vi "aal_moving average with decimation by order (real input).vi"(1 "Reset":bool, 2 "N":i32=2, 3 "x":dbl[](array[numeric])) -> (0 "y":dbl[](array[numeric]))   [LabVIEW 2014, in "NI_AALPro.lvlib"]
uses:
  NI_AALPro.lvlib
  lvanlys.dll
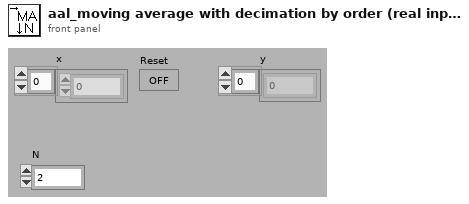
[diagram p1: front panel]
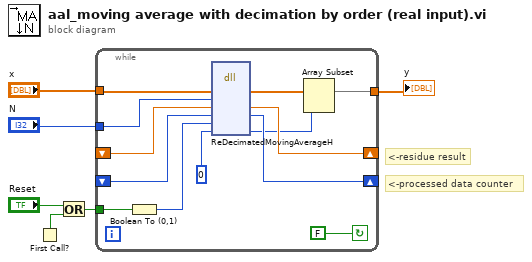
[diagram p0: block diagram]
diagram:
  # "<-residue result"
  # "<-processed data counter"
  n1 = First Call?() -> (First Call?: T/F=w3:bool)
  n2 = Or(x="Reset", y=w3) -> (x .or. y?=w4:bool)
  n3 = while {
    tunnel: [w16] -> w1
    tunnel: "N" -> [w14]
    tunnel: w4 -> [w19]
    tunnel: "x" -> [w18]
    shift-left: _ -> [w11]
    shift-right: [w10] -> _
    shift-left: _ -> [w13]
    shift-right: [w12] -> _
    stop <- FALSE continue-if-true
    n4 = Boolean To (0,1)(Boolean=w19) -> (0, 1=w9:i16)
    n5 = dll-call lib="C:/Program Files (x86)/National Instruments/LabVIEW 2014/resource/lvanlys.*" fn="ReDecimatedMovingAverageH"("x"=w18, "N"=w14, "state"=w13, "cnt"=w11, "reset"=w9, "out_len"=0 ("yH")) -> ("x"=w17:dbl[], "state"=w12:dbl, "cnt"=w10:i32, "out_len"=w7:i32)  [unwired: 6 in, 2 out]
    n6 = Array Subset(array=w17, length=w7) -> (w16:dbl[])  [unwired: 1 in]
  }
  "y" <- w1
